vi "PDU GUI Configure.vi"(8 "error in (no error)":errorcluster, 11 "Power Distribution in":refnum<class "Power Distribution.lvclass">) -> (0 "error out":errorcluster, 3 "Power Distribution out":refnum<class "Power Distribution.lvclass">)   [LabVIEW 2022 SP3, in "Power Distribution.lvclass"]
uses:
  Power Distribution.lvclass
  Power Distribution.lvclass/Power Distribution.ctl
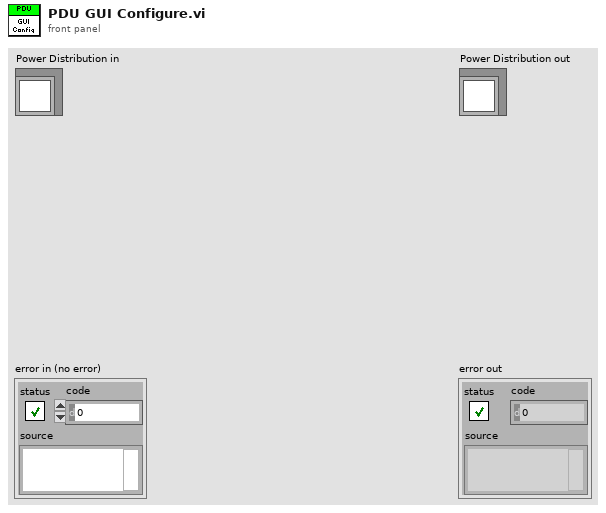
[diagram p1: front panel]
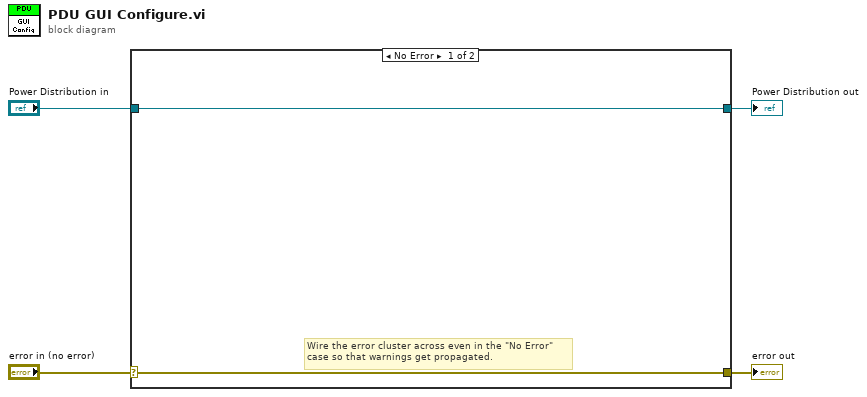
[diagram p0: block diagram]
diagram:
  n1 = case shown="No Error" "error in (no error)" {
    selector: "error in (no error)" -> [w6 w8]
    tunnel: [w6 w8] -> w3
    tunnel: [w5 w7] -> w1
    tunnel: "Power Distribution in" -> [w5 w7]
    frame No Error {
      # "Wire the error cluster across even in the \"No Error\"\ncase so that warnings get propagated."
    }
    frame Error {
    }
  }
  "error out" <- w3
  "Power Distribution out" <- w1
